vi "time_parse_weather.vi"(1 "Current Time":timestamp) -> (13 "Fractional Seconds":dbl, 14 "Year":u32, 15 "Month":u32, 16 "Day":u32, 17 "Hour":u32, 18 "Minutes":u32, 19 "Seconds":u32)   [LabVIEW 2018]
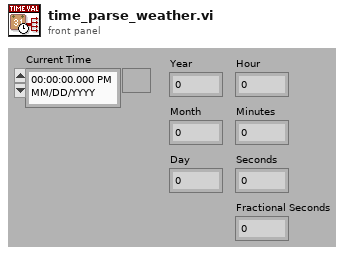
[diagram p1: front panel]
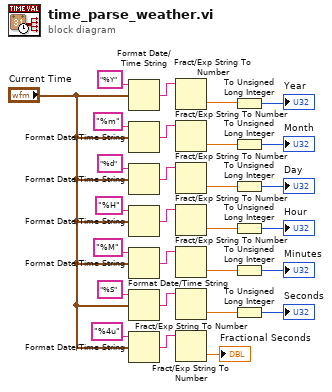
[diagram p0: block diagram]
diagram:
  n1 = Format Date/Time String(time format string (%c)="%Y", seconds (now)="Current Time") -> (date/time string=w27:string)  [unwired: 1 in]
  n2 = Format Date/Time String(time format string (%c)="%m", seconds (now)="Current Time") -> (date/time string=w25:string)  [unwired: 1 in]
  n3 = Format Date/Time String(time format string (%c)="%d", seconds (now)="Current Time") -> (date/time string=w22:string)  [unwired: 1 in]
  n4 = Format Date/Time String(time format string (%c)="%H", seconds (now)="Current Time") -> (date/time string=w24:string)  [unwired: 1 in]
  n5 = Format Date/Time String(time format string (%c)="%M", seconds (now)="Current Time") -> (date/time string=w15:string)  [unwired: 1 in]
  n6 = Format Date/Time String(time format string (%c)="%S", seconds (now)="Current Time") -> (date/time string=w17:string)  [unwired: 1 in]
  n7 = Format Date/Time String(time format string (%c)="%4u", seconds (now)="Current Time") -> (date/time string=w19:string)  [unwired: 1 in]
  n8 = Fract/Exp String To Number(string=w27) -> (number=w6:dbl)  [unwired: 3 in, 1 out]
  n9 = Fract/Exp String To Number(string=w25) -> (number=w5:dbl)  [unwired: 3 in, 1 out]
  n10 = Fract/Exp String To Number(string=w22) -> (number=w4:dbl)  [unwired: 3 in, 1 out]
  n11 = Fract/Exp String To Number(string=w24) -> (number=w3:dbl)  [unwired: 3 in, 1 out]
  n12 = Fract/Exp String To Number(string=w15) -> (number=w2:dbl)  [unwired: 3 in, 1 out]
  n13 = Fract/Exp String To Number(string=w17) -> (number=w1:dbl)  [unwired: 3 in, 1 out]
  n14 = Fract/Exp String To Number(string=w19) -> (number=→"Fractional Seconds":dbl)  [unwired: 3 in, 1 out]
  n15 = To Unsigned Long Integer(number=w6) -> (unsigned 32bit integer=→"Year":u32)
  n16 = To Unsigned Long Integer(number=w5) -> (unsigned 32bit integer=→"Month":u32)
  n17 = To Unsigned Long Integer(number=w4) -> (unsigned 32bit integer=→"Day":u32)
  n18 = To Unsigned Long Integer(number=w3) -> (unsigned 32bit integer=→"Hour":u32)
  n19 = To Unsigned Long Integer(number=w2) -> (unsigned 32bit integer=→"Minutes":u32)
  n20 = To Unsigned Long Integer(number=w1) -> (unsigned 32bit integer=→"Seconds":u32)
